vi "Add Initialization Block Diagram Content.vi"(8 "error in (no error)":errorcluster, 10 "Init":T1, 11 "Module in":refnum<class "Module.lvclass">) -> (0 "error out":errorcluster, 3 "Module out":refnum<class "Module.lvclass">)   [LabVIEW 2025, in "Module.lvclass"]
doc: "Iterate through all signals and dynamically generate IP in the main init structure."
uses:
  Module.lvclass
  VI/VI/Init.Refs.ctl
  <vilib>/Utility/miscctls.llb/LVPointTypeDef.ctl
  Module.lvclass/Module.ctl
  VI/VI/Error Codes.ctl
  Signal/Signal/Read IO Name.vi
  Signal/Signal/Read Signal Name.vi
  Signal/Signal/Signal.lvclass
  VI/VI/VI.lvclass
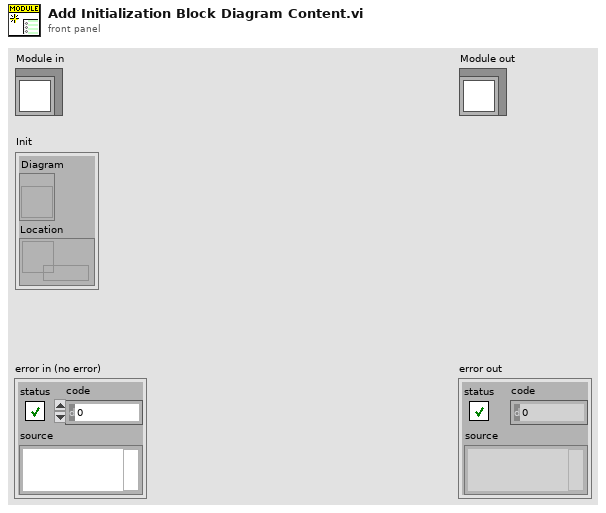
[diagram p1: front panel]
types:
  T1 = typedef "VI.lvclass/Init.Refs.ctl" = cluster{"Diagram":refnum<vi>, "Location":refnum<data-value>}
  T2 = typedef "VI.lvclass/Error Codes.ctl" = enum16{"Signal Unsupported", "Module Unsupported", "Parameter Unsupported", "Signal Code Gen Error", "Module Code Gen Error", "Cleanup Code Error", "Signal Direction Mismatch", "Signal Type Mismatch", "Module Channel Number Mismatch", "Minimum Channels Mismatch"}
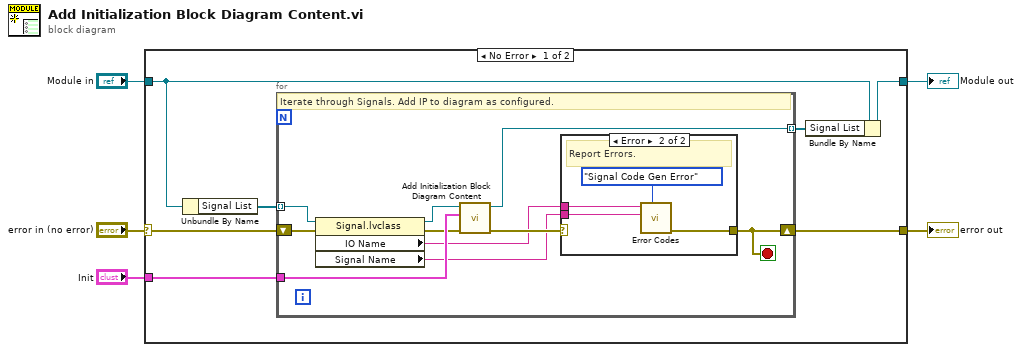
[diagram p0: block diagram]
diagram:
  n1 = case shown="No Error" "error in (no error)" {
    selector: "error in (no error)" -> [w8 w29]
    tunnel: [w11 w29] -> w4
    tunnel: [w9 w28] -> w2
    tunnel: "Module in" -> [w7 w28]
    tunnel: "Init" -> [w12 _]
    frame No Error {
      n2 = Unbundle By Name(w7) -> ("Signal List"=w6:refnum<class "Signal.lvclass">[])
      n3 = for {
        shift-right: [w15] -> w11
        shift-left: w8 -> [w18]
        tunnel: w12 -> [w22]
        tunnel: [w21] -> w10 mode=indexing
        tunnel: w6 -> [w20] mode=indexing
        stop <- w15 stop-if-true
        # "Iterate through Signals. Add IP to diagram as configured."
        n4 = property class="Signal.lvclass"(reference=w20, error in=w18) -> (reference out=w19:refnum<class "Signal.lvclass">, error out=w17:errorcluster, "IO Name"=w14:string, "Signal Name"=w13:string)
        n5 = call-dynamic "Add Initialization Block Diagram Content.vi"("error in (no error)"=w17, "Init"=w22, "IO Class in"=w19) -> ("error out"=w16:errorcluster, "IO Class out"=w21:refnum<class "Signal.lvclass">)  [unwired: 7 in]
        n6 = case shown="Error" w16 {
          selector: w16 -> [w23 _]
          tunnel: [w23 w26] -> w15
          tunnel: w14 -> [_ w25]
          tunnel: w13 -> [_ w24]
          frame No Error {
          }
          frame Error {
            # "Report Errors."
            n7 = call "Error Codes.vi"("Error"=Error_Codes."Signal Code Gen Error", "Module/Signal Name"=w24, "Module/Signal Resource"=w25) -> ("error out"=w26:errorcluster)  [unwired: 8 in]
          }
        }
      }
      n8 = Bundle By Name(cluster=w7, "Signal List"=w10) -> (w9:refnum<class "Module.lvclass">)
    }
    frame Error {
    }
  }
  "error out" <- w4
  "Module out" <- w2
